vi "Main.vi"(11 "Module Admin":refnum<class "Delacor_lib_QMH_Module Admin.lvclass">) -> ()   [LabVIEW 2024, in "MoneyControl.lvlib"]
doc: "This template is based off of the Queued Message Handler design pattern and the Queued Message Handler project template that ships with LabVIEW.\n\nThe main difference is that the queue is private to this module and communication between modules is performed via Broadcast and Request events.\n\nRequest events are wrapped in public API methods and are handled in the Event Handling Loop (EHL) of this VI. Any module can register for Broadcast events sent by this module. The EHL generates messages based on user interface actions.\n\nThe Message Handling Loop (MHL) processes messages generated by the EHL, or by other messages. The messages are string values, so new messages can be added easily to the Message Cases case structure in the MHL. Each message cluster can also provide an optional value for Message Data, which is a variant that can be converted to whatever message-specific data is required.\n_____\nBased on DQMH Dev Tools: Project Template 7.1.0.1503."
uses:
  MoneyControl.lvlib
  <vilib>/Delacor/Delacor QMH/Libraries/Module Admin_class/Delacor_lib_QMH_Module Admin.lvclass
  Module Data--cluster.ctl
  <vilib>/Utility/miscctls.llb/LVFontTypeDef.ctl
  Stop Argument--cluster.ctl
  <vilib>/Delacor/Delacor QMH/Libraries/Message Queue_class/Delacor_lib_QMH_Message Queue.lvclass/Delacor_lib_QMH_Message Queue.ctl
  <vilib>/Delacor/Delacor QMH/Libraries/Module Admin_class/Delacor_lib_QMH_Module Admin.lvclass/Delacor_lib_QMH_Module Admin.ctl
  Draw FP in Subpanel Argument--cluster.ctl
  Remove From Subpanel Argument--cluster.ctl
  Incrementa Credito Argument--cluster.ctl
  Cancelar Argument--cluster.ctl
  <vilib>/Delacor/Delacor QMH/Libraries/Message Queue_class/Delacor_lib_QMH_Enqueue Message (Single).vi
  <vilib>/Delacor/Delacor QMH/Libraries/Module Admin_class/Delacor_lib_QMH_Get External Launch.vi
  <vilib>/Delacor/Delacor QMH/Libraries/Message Queue_class/Delacor_lib_QMH_Message Queue.lvclass
  <vilib>/PantherLAB/Message Module/Libraries/Message/PantherLAB_lib_Message.lvlib
panel:
  in  "Moneda 1":bool caption="1"
  in  "Moneda 5":bool caption="5"
  in  "Moneda 2":bool caption="2"
  out "error out":errorcluster
  out "Status":string
  in  "Moneda 10":bool caption="10"
  in  "Cancelar":bool
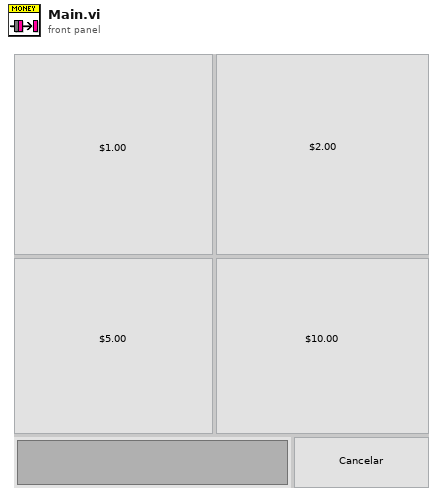
[diagram p1: front panel]
types:
  T1 = typedef "MoneyControl.lvlib/Request Events--cluster.ctl" = cluster{"Stop Module":refnum<user-event>, "Show Panel":refnum<user-event>, "Hide Panel":refnum<user-event>, "Get Module Execution Status":refnum<user-event>, "Show Diagram":refnum<user-event>, "Draw FP in Subpanel":refnum<user-event>, "Remove From Subpanel":refnum<user-event>, "Incrementa Credito":refnum<user-event>, "Cancelar":refnum<user-event>}
  T2 = typedef "PantherLAB_lib_Message.lvlib/Broadcast Events--cluster.ctl" = cluster{"Module Did Init":refnum<user-event>, "Status Updated":refnum<user-event>, "Error Reported":refnum<user-event>, "Module Did Stop":refnum<user-event>, "Update Module Execution Status":refnum<user-event>}
  T3 = typedef "MoneyControl.lvlib/Module Data--cluster.ctl" = cluster{"Status":string, "Sub Panel":refnum<vi>, "Credito":dbl}
  T4 = typedef "LVFontTypeDef.ctl" = cluster{"Font Name":string, "Size":u16, "Bold":bool, "Italic":bool, "Underline":bool, "Strikeout":bool, "Color":u32}
  T5 = enum32{"invalid lock state", "Not Locked", "Locked (No Password)", "Password-protected"}
  T6 = typedef "MoneyControl.lvlib/Stop Argument--cluster.ctl" = cluster{"Origin":string, "Exit via Stop Module Req?":bool, "Wait for Module to stop?":bool}
  T7 = typedef "MoneyControl.lvlib/Draw FP in Subpanel Argument--cluster.ctl" = cluster{"Sub Panel":refnum<vi>}
  T8 = typedef "MoneyControl.lvlib/Remove From Subpanel Argument--cluster.ctl" = cluster{"Boolean":bool}
  T9 = typedef "MoneyControl.lvlib/Incrementa Credito Argument--cluster.ctl" = cluster{"Credito":dbl}
  T10 = typedef "MoneyControl.lvlib/Cancelar Argument--cluster.ctl" = cluster{"Boolean":bool}
  T11 = enum32{"Invalid", "Standard", "Closed", "Hidden", "Minimized", "Maximized"}
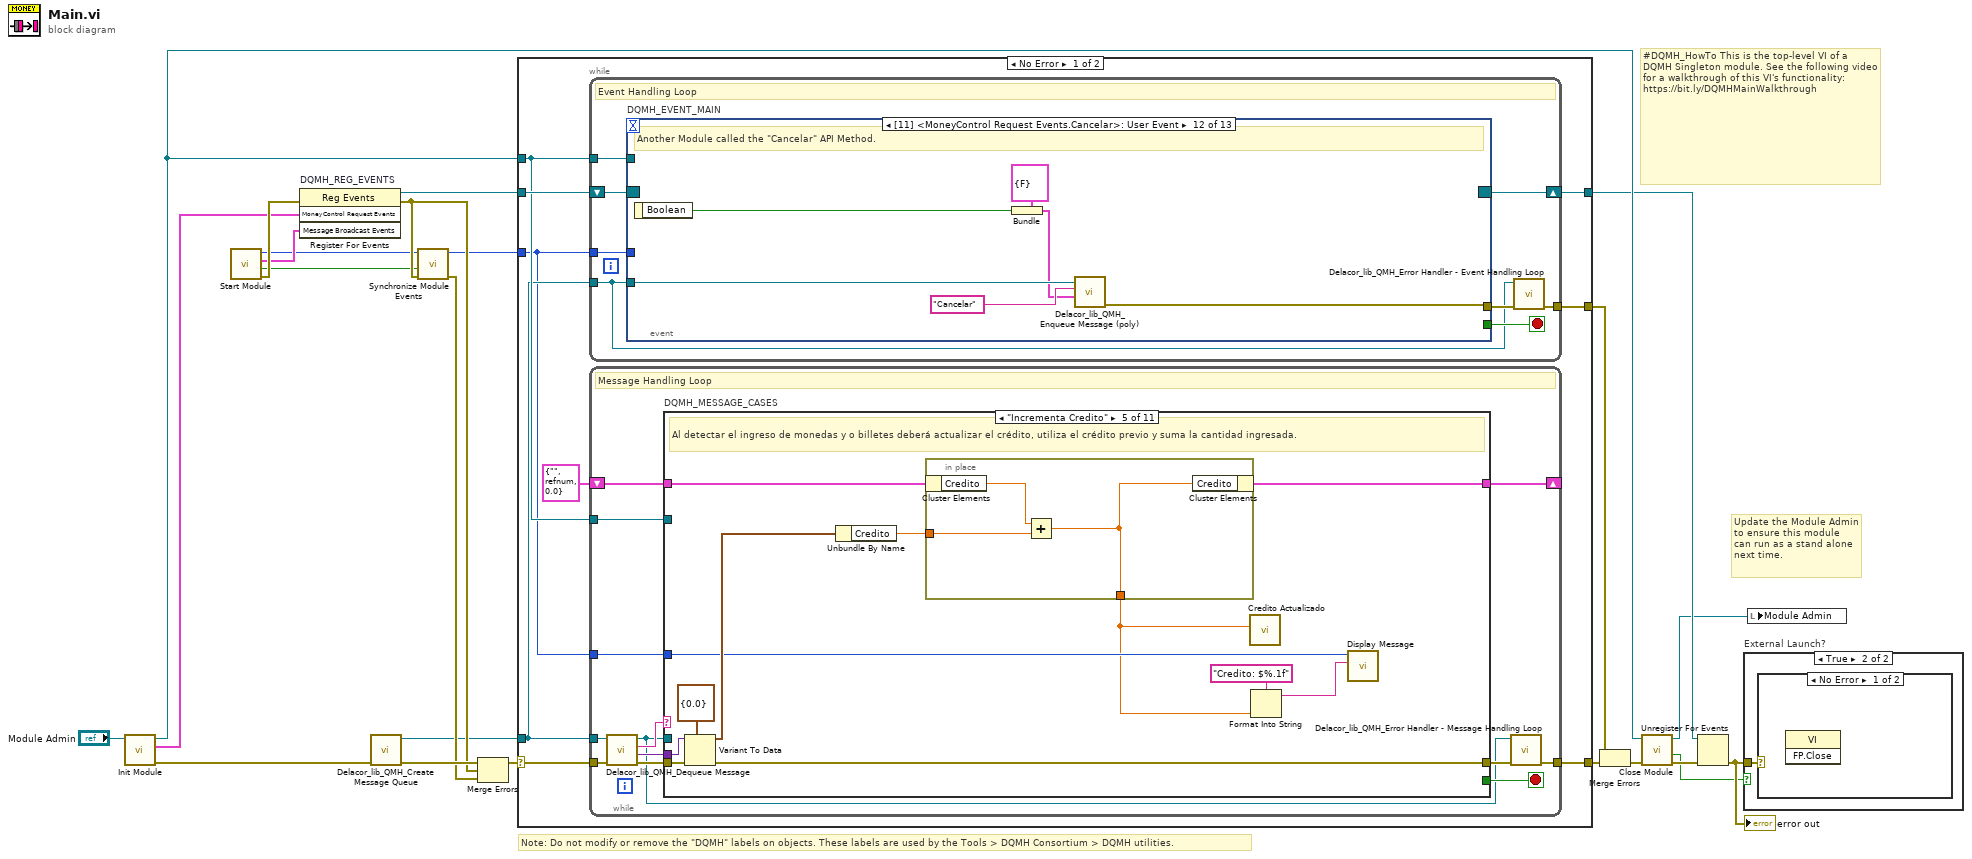
[diagram p0: block diagram]
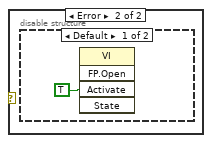
[diagram p3: hidden frame]
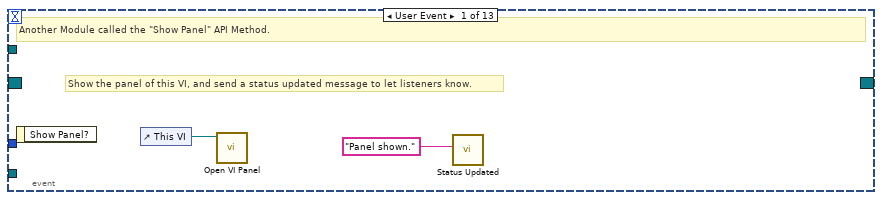
[diagram p5: hidden frame]
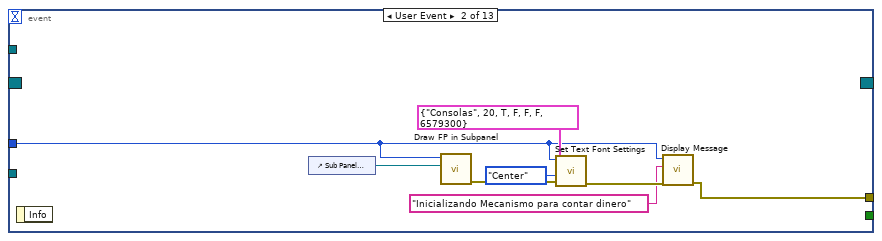
[diagram p6: hidden frame]
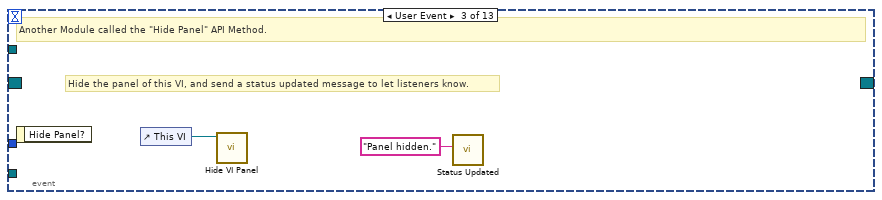
[diagram p7: hidden frame]
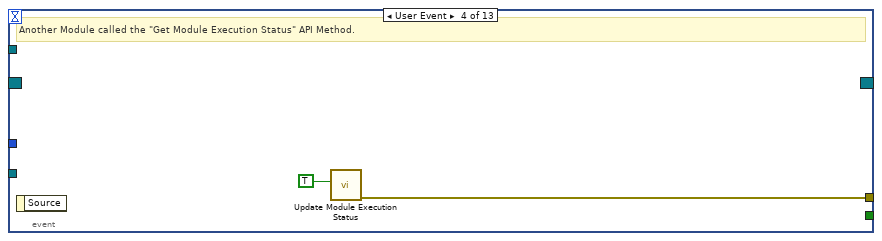
[diagram p8: hidden frame]
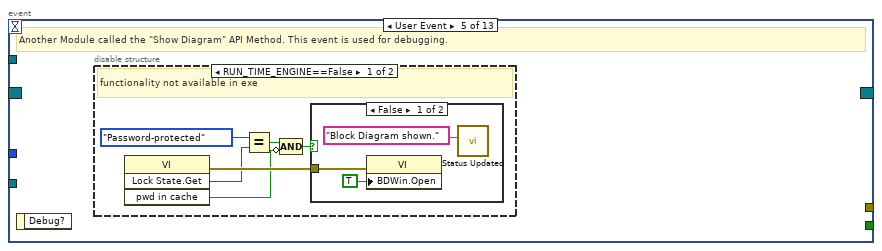
[diagram p9: hidden frame]
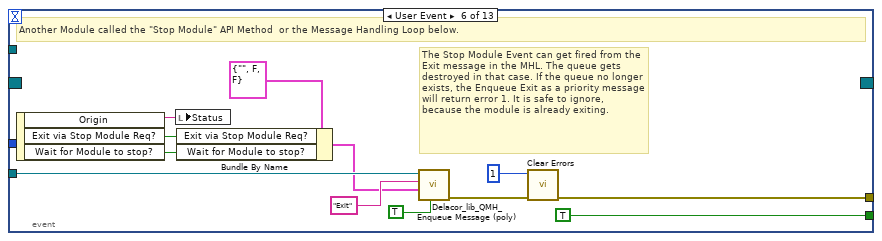
[diagram p12: hidden frame]
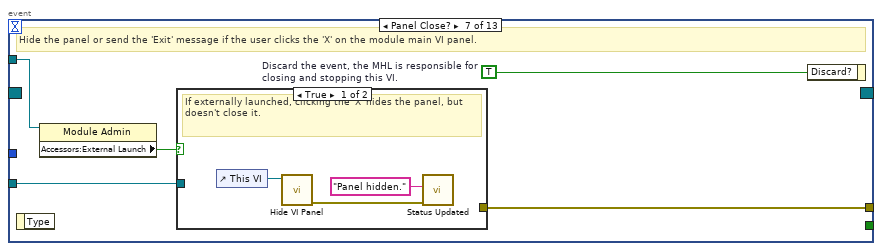
[diagram p13: hidden frame]
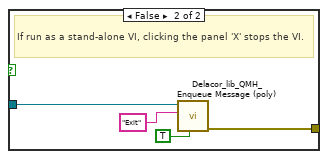
[diagram p14: hidden frame]
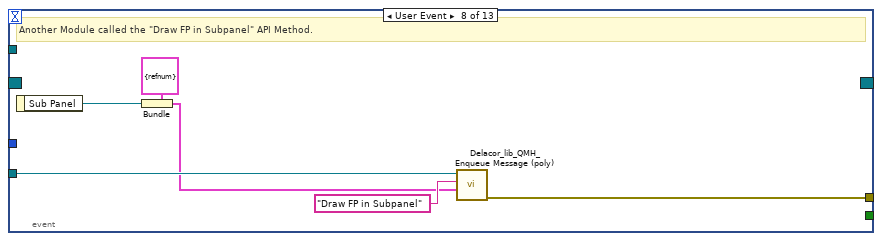
[diagram p15: hidden frame]
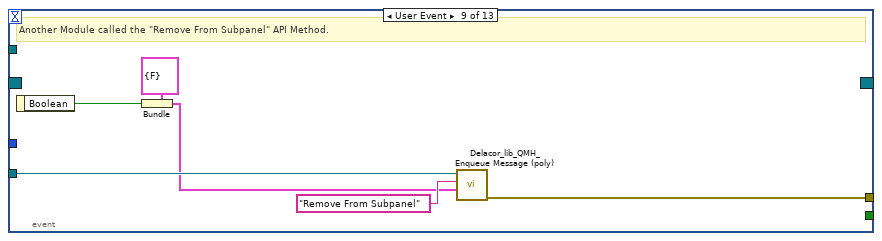
[diagram p16: hidden frame]
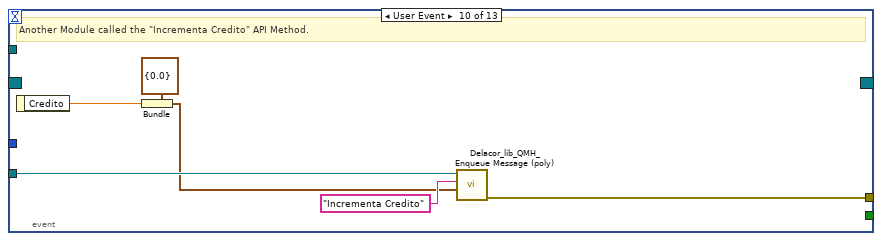
[diagram p17: hidden frame]
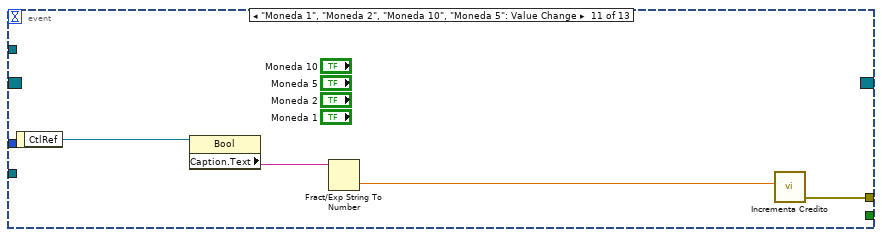
[diagram p18: hidden frame]
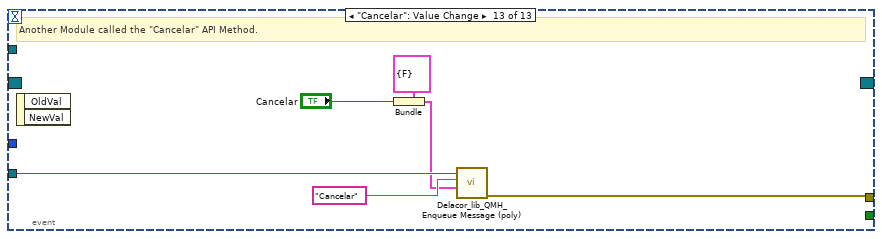
[diagram p19: hidden frame]
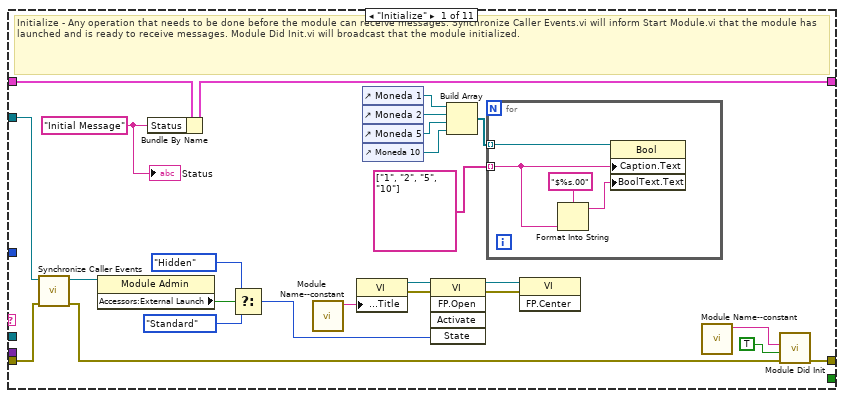
[diagram p20: hidden frame]
diagram:
  # "#DQMH_HowTo This is the top-level VI of a DQMH Singleton module. See the following video for a walkthrough of this VI's functionality: https://bit.ly/DQMHMainWalkthrough"
  # "Note: Do not modify or remove the \"DQMH\" labels on objects. These labels are used by the Tools > DQMH Consortium > DQMH utilities."
  # "Update the Module Admin to ensure this module can run as a stand alone next time."
  n1 = call "Init Module.vi"("Singleton Module Admin in"="Module Admin") -> ("error out"=w22:errorcluster, "MoneyControl Request Events"=w9:T1, "Singleton Module Admin out"=w12:refnum<class "Delacor_lib_QMH_Module Admin.lvclass">)  [unwired: 8 in]
  n2 = call <vilib>:"Start Module.vi"() -> ("error out"=w13:errorcluster, "Wait for Event Sync?"=w2:bool, "Message Broadcast Events"=w4:T2, "Module ID"=w3:i32)  [unwired: 7 in, 1 out]
  n3 = register-events "DQMH_REG_EVENTS"(error in=w13, w9, w4) -> (reference out=w10:refnum<event-registration>, error out=w15:errorcluster)  [unwired: 1 in]
  n4 = call <vilib>:"Delacor_lib_QMH_Create Message Queue.vi"("error in"=w22) -> ("error out"=w17:errorcluster, "Message Queue"=w8:refnum<class "Delacor_lib_QMH_Message Queue.lvclass">)  [unwired: 9 in]
  n5 = call <vilib>:"Synchronize Module Events.vi"("error in"=w15, "Wait for Event Sync?"=w2, "Module ID in"=w3) -> ("error out"=w14:errorcluster, "Module ID out"=w1:i32)  [unwired: 7 in]
  n6 = Merge Errors(w17, w15, w14) -> (w16:errorcluster)
  n7 = case shown="No Error" w16 {
    selector: w16 -> [w30 w292]
    tunnel: [w32 w291] -> w23
    tunnel: [w29 w290] -> w11
    tunnel: w10 -> [w27 w290]
    tunnel: w8 -> [w25 w286]
    tunnel: [w31 _] -> w20
    tunnel: w12 -> [w26 w287]
    tunnel: w1 -> [w24 w284]
    frame No Error {
      n8 = while {
        tunnel: w25 -> [w34]
        shift-right: [w37] -> w29
        shift-left: w27 -> [w38]
        tunnel: [w39] -> w31
        tunnel: w26 -> [w35]
        tunnel: w24 -> [w33]
        stop <- w36 stop-if-true
        # "Event Handling Loop"
        n9 = event "DQMH_EVENT_MAIN" shown="[11] <MoneyControl Request Events.Cancelar>: User Event" {
          selector: w38 -> [_ _ _ _ _ _ _ _ _ _ _ _ _]
          dyn-events: [_ _ _ _ _ _ _ _ _ _ _ _ _] -> w37
          timeout: _ -> [_ _ _ _ _ _ _ _ _ _ _ _ _]
          tunnel: [_ _ _ _ _ TRUE ("Discard?") _ _ _ _ _ _ _] -> w36
          tunnel: w34 -> [_ _ _ _ _ w71 w78 w92 w98 w104 _ w115 w121]
          tunnel: [_ w48 _ w54 _ w74 w80 w93 w99 w105 w109 w110 w117] -> w40
          tunnel: w35 -> [_ _ _ _ _ _ w77 _ _ _ _ _ _]
          tunnel: w33 -> [_ w44 _ _ _ _ _ _ _ _ _ _ _]
          event User Event {
            # "Show the panel of this VI, and send a status updated message to let listeners know."
            # "Another Module called the \"Show Panel\" API Method."
            n10 = event-data() -> ()  [unwired: 1 in, 1 out]
            n11 = control-ref of="This VI"() -> (w42:refnum<vi>)
            n12 = call "Open VI Panel.vi"("VI"=w42) -> ()  [unwired: 10 in, 1 out]
            n13 = call "Status Updated.vi"("Status"="Panel shown." ("format string")) -> ()  [unwired: 10 in, 1 out]
          }
          event User Event {
            n14 = event-data() -> ()  [unwired: 1 in, 1 out]
            n15 = control-ref of="Sub Panel Mensajes"() -> (w47:refnum<vi>)
            n16 = call <vilib>:"Draw FP in Subpanel.vi"("Sub Panel"=w47, "Module ID"=w44) -> ("error out"=w50:errorcluster)  [unwired: 9 in]
            n17 = call <vilib>:"Set Text Font Settings.vi"("error in"=w50, "Text.Justification"=enum16{"Left", "Center", "Right"}."Center", "Font"=T4 {"Font Name"="Consolas", "Size"=20, "Bold"=TRUE, "Italic"=FALSE, "Underline"=FALSE, "Strikeout"=FALSE, "Color"=6579300}, "Module ID"=w44) -> ("error out"=w49:errorcluster)  [unwired: 7 in]
            n18 = call <vilib>:"Display Message.vi"("error in"=w49, "Message"="Inicializando Mecanismo para contar dinero", "Module ID"=w44) -> ("error out"=w48:errorcluster)  [unwired: 8 in]
          }
          event User Event {
            # "Hide the panel of this VI, and send a status updated message to let listeners know."
            # "Another Module called the \"Hide Panel\" API Method."
            n19 = event-data() -> ()  [unwired: 1 in, 1 out]
            n20 = control-ref of="This VI"() -> (w52:refnum<vi>)
            n21 = call "Hide VI Panel.vi"("VI"=w52) -> ()  [unwired: 10 in, 1 out]
            n22 = call "Status Updated.vi"("Status"="Panel hidden." ("format string")) -> ()  [unwired: 10 in, 1 out]
          }
          event User Event {
            # "Another Module called the \"Get Module Execution Status\" API Method."
            n23 = event-data() -> ()  [unwired: 1 in, 1 out]
            n24 = call "Update Module Execution Status.vi"("Running?"=TRUE) -> ("error out"=w54:errorcluster)  [unwired: 10 in]
          }
          event User Event {
            # "Another Module called the \"Show Diagram\" API Method. This event is used for debugging."
            n25 = event-data() -> ()  [unwired: 1 in, 1 out]
            n26 = disable-structure shown="RUN_TIME_ENGINE==False" {
              frame condition #0 (active) {
                # "functionality not available in exe"
                n27 = invoke on="Invoke Node" class="VI" method="Lock State.Get"() -> (error out=w60:errorcluster, "Get Lock State"=w59:T5, "pwd in cache"=w56:bool)  [unwired: 4 in, 1 out]
                n28 = Equal?(x=T5."Password-protected", y=w59) -> (x = y?=w57:bool)
                n29 = Compound Arithmetic op=AND(w57, invert w56) -> (w55:bool)
                n30 = case shown="False" w55 {
                  tunnel: w60 -> [w63 _]
                  frame False {
                    n31 = property on="Property Node" class="VI"(error in=w63, "BDWin.Open"=TRUE ("Block Diagram Window:Open")) -> ()  [unwired: 1 in, 2 out]
                    n32 = call "Status Updated.vi"("Status"="Block Diagram shown." ("format string")) -> ()  [unwired: 10 in, 1 out]
                  }
                  frame True {
                    # "Password-protected VI, and the password is not in the cache. Do not show the diagram."
                  }
                }
              }
              frame condition #1 {
              }
            }
          }
          event User Event {
            # "The Stop Module Event can get fired from the Exit message in the MHL. The queue gets destroyed in that case. If the queue no longer exists, the Enqueue Exit as a priority message will return error 1. It is safe to ignore, because the module is already exiting."
            # "Another Module called the \"Stop Module\" API Method  or the Message Handling Loop below."
            n33 = event-data() -> ("Origin"=w70:string, "Exit via Stop Module Req?"=w66:bool, "Wait for Module to stop?"=w65:bool)  [unwired: 1 in]
            n34 = local write "Status"(w70) -> ()
            n35 = Bundle By Name(cluster=T6 {"Origin"="", "Exit via Stop Module Req?"=FALSE, "Wait for Module to stop?"=FALSE} ("Stop Argument"), "Exit via Stop Module Req?"=w66, "Wait for Module to stop?"=w65) -> (w64:T6)
            n36 = call-poly <vilib>:"Delacor_lib_QMH_Enqueue Message (poly).vi"("Priority Message? (F)"=TRUE, "Message Data"=w64, "Message"="Exit", "Message Queue in"=w71) -> ("error out"=w75:errorcluster)  [unwired: 6 in, 1 out]
            n37 = call <vilib>:"Clear Errors.vi"("error in (no error)"=w75, "specific error code to clear (0: all)"=1) -> ("error out"=w74:errorcluster)  [unwired: 4 in, 1 out]
          }
          event Panel Close? {
            w79 = TRUE  # Discard the event, the MHL is responsible for closing and stopping this VI.
            # "Hide the panel or send the 'Exit' message if the user clicks the 'X' on the module main VI panel."
            n38 = event-data() -> ()  [unwired: 1 in, 1 out]
            n39 = property on="Property Node" class="Module Admin"(reference=w77) -> ("Accessors:External Launch"=w76:bool)  [unwired: 1 in, 2 out]
            n40 = case shown="True" w76 {
              tunnel: w78 -> [_ w86]
              tunnel: [_ w87] -> w80
              frame True {
                # "If externally launched, clicking the 'X' hides the panel, but doesn't close it."
                n41 = control-ref of="This VI"() -> (w82:refnum<vi>)
                n42 = call "Hide VI Panel.vi"("VI"=w82) -> ("error out"=w83:errorcluster)  [unwired: 10 in]
                n43 = call "Status Updated.vi"("error in"=w83, "Status"="Panel hidden." ("format string")) -> ()  [unwired: 9 in, 1 out]
              }
              frame False {
                # "If run as a stand-alone VI, clicking the panel 'X' stops the VI."
                n44 = call-poly <vilib>:"Delacor_lib_QMH_Enqueue Message (poly).vi"("Priority Message? (F)"=TRUE, "Message"="Exit", "Message Queue in"=w86) -> ("error out"=w87:errorcluster)  [unwired: 7 in, 1 out]
              }
            }
            n45 = event-data ("Event Filter Node")("Discard?"=w79) -> ()  [unwired: 1 in, 1 out]
          }
          event User Event {
            # "Another Module called the \"Draw FP in Subpanel\" API Method."
            n46 = event-data() -> ("Sub Panel"=w88:refnum<vi>)  [unwired: 1 in]
            n47 = Bundle(cluster=T7 {"Sub Panel"=refnum} ("Draw FP in Subpanel Argument"), "Sub Panel"=w88) -> (w89:T7)
            n48 = call-poly <vilib>:"Delacor_lib_QMH_Enqueue Message (poly).vi"("Message Data"=w89, "Message"="Draw FP in Subpanel", "Message Queue in"=w92) -> ("error out"=w93:errorcluster)  [unwired: 7 in, 1 out]
          }
          event User Event {
            # "Another Module called the \"Remove From Subpanel\" API Method."
            n49 = event-data() -> ("Boolean"=w94:bool)  [unwired: 1 in]
            n50 = Bundle(cluster=T8 {"Boolean"=FALSE} ("Remove From Subpanel Argument"), "Boolean"=w94) -> (w95:T8)
            n51 = call-poly <vilib>:"Delacor_lib_QMH_Enqueue Message (poly).vi"("Message Data"=w95, "Message"="Remove From Subpanel", "Message Queue in"=w98) -> ("error out"=w99:errorcluster)  [unwired: 7 in, 1 out]
          }
          event User Event {
            # "Another Module called the \"Incrementa Credito\" API Method."
            n52 = event-data() -> ("Credito"=w100:dbl)  [unwired: 1 in]
            n53 = Bundle(cluster=T9 {"Credito"=0.0} ("Incrementa Credito Argument"), "Credito"=w100) -> (w101:T9)
            n54 = call-poly <vilib>:"Delacor_lib_QMH_Enqueue Message (poly).vi"("Message Data"=w101, "Message"="Incrementa Credito", "Message Queue in"=w104) -> ("error out"=w105:errorcluster)  [unwired: 7 in, 1 out]
          }
          event "Moneda 1", "Moneda 2", "Moneda 10", "Moneda 5": Value Change {
            n55 = event-data() -> ("CtlRef"=w108:refnum<vi>)  [unwired: 1 in]
            n56 = property class="Bool"(reference=w108) -> ("Caption.Text"=w107:string)  [unwired: 1 in, 2 out]
            n57 = Fract/Exp String To Number(string=w107) -> (number=w106:dbl)  [unwired: 3 in, 1 out]
            n58 = call "Incrementa Credito.vi"("Credito"=w106) -> ("error out"=w109:errorcluster)  [unwired: 10 in]
          }
          event User Event {
            # "Another Module called the \"Cancelar\" API Method."
            n59 = event-data() -> ("Boolean"=w111:bool)  [unwired: 1 in]
            n60 = Bundle(cluster=T10 {"Boolean"=FALSE} ("Cancelar Argument"), "Boolean"=w111) -> (w112:T10)
            n61 = call-poly <vilib>:"Delacor_lib_QMH_Enqueue Message (poly).vi"("Message Data"=w112, "Message"="Cancelar", "Message Queue in"=w115) -> ("error out"=w110:errorcluster)  [unwired: 7 in, 1 out]
          }
          event "Cancelar": Value Change {
            # "Another Module called the \"Cancelar\" API Method."
            n62 = event-data() -> ()  [unwired: 1 in, 2 out]
            n63 = Bundle(cluster=T10 {"Boolean"=FALSE} ("Cancelar Argument"), "Boolean"="Cancelar") -> (w118:T10)
            n64 = call-poly <vilib>:"Delacor_lib_QMH_Enqueue Message (poly).vi"("Message Data"=w118, "Message"="Cancelar", "Message Queue in"=w121) -> ("error out"=w117:errorcluster)  [unwired: 7 in, 1 out]
          }
        }
        n65 = call-dynamic "Delacor_lib_QMH_Error Handler - Event Handling Loop.vi"("error in"=w40, "Message Queue in"=w34) -> ("dup error in"=w39:errorcluster)  [unwired: 8 in, 1 out]
      }
      n66 = while {
        tunnel: w25 -> [w123]
        shift-right: [w129] -> _
        shift-left: T3 {"Status"="", "Sub Panel"=refnum, "Credito"=0.0} ("Data Cluster") -> [w130]
        tunnel: w30 -> [w134]
        tunnel: [w132] -> w32
        tunnel: w26 -> [w125]
        tunnel: w24 -> [w122]
        stop <- w128 stop-if-true
        # "Message Handling Loop"
        n67 = call-dynamic "Delacor_lib_QMH_Dequeue Message.vi"("error in"=w134, "Message Queue in"=w123) -> ("error out"=w133:errorcluster, "Message Data"=w126:variant, "Message"=w127:string, "Message Queue out"=w124:refnum<class "Delacor_lib_QMH_Message Queue.lvclass">)  [unwired: 6 in]
        n68 = case "DQMH_MESSAGE_CASES" shown="\"Incrementa Credito\"" w127 {
          selector: w127 -> [_ _ _ _ _ _ _ _ _ _ w279]
          tunnel: w124 -> [_ _ _ _ _ _ _ _ w242 w267 _]
          tunnel: w133 -> [w157 w165 w181 w199 w217 w232 w237 w239 w250 w273 w282]
          tunnel: [w155 w165 w180 w197 w216 w231 w236 w239 w246 w268 w283] -> w131
          tunnel: w130 -> [w146 w164 w176 w193 w212 w227 w235 w238 w244 w259 w280]
          tunnel: [w145 w164 w172 w190 w211 w226 w235 w238 w244 w259 w280] -> w129
          tunnel: [_ _ _ _ _ _ _ _ _ w266 _] -> w128
          tunnel: w126 -> [_ _ w175 w196 w215 w230 _ _ w243 w265 _]
          tunnel: w125 -> [w147 _ _ _ _ _ _ _ w241 w260 _]
          tunnel: w122 -> [_ _ _ _ w209 w224 _ _ _ w257 _]
          frame "Initialize" {
            w141 = "Initial Message" ("Initial Message")
            # "Initialize - Any operation that needs to be done before the module can receive messages. Synchronize Caller Events.vi will inform Start Module.vi that the module has launched and is ready to receive messages. Module Did Init.vi will broadcast that the module initialized."
            n69 = call "Synchronize Caller Events.vi"("error in"=w157, "Singleton Module Admin in"=w147) -> ("error out"=w156:errorcluster, "Singleton Module Admin out"=w142:refnum<class "Delacor_lib_QMH_Module Admin.lvclass">)  [unwired: 8 in]
            n70 = property on="Property Node" class="Module Admin"(reference=w142) -> ("Accessors:External Launch"=w151:bool)  [unwired: 1 in, 2 out]
            n71 = Bundle By Name(cluster=w146, "Status"=w141) -> (w145:T3)
            n72 = Select(t=T11."Hidden" ("State"), s=w151, f=T11."Standard" ("State")) -> (s? t:f=w148:T11)
            n73 = call "Module Name--constant.vi"() -> ("Module Name"=w154:string)  [unwired: 11 in]
            n74 = property on="Property Node" class="VI"("Front Panel.Title"=w154) -> (reference out=w153:refnum<vi>, error out=w159:errorcluster)  [unwired: 2 in]
            n75 = control-ref of="Moneda 1"() -> (w140:refnum<vi>)
            n76 = control-ref of="Moneda 2"() -> (w139:refnum<vi>)
            n77 = control-ref of="Moneda 5"() -> (w138:refnum<vi>)
            n78 = control-ref of="Moneda 10"() -> (w137:refnum<vi>)
            n79 = invoke on="Invoke Node" class="VI" method="FP.Open"(reference=w153, error in=w159, "State"=w148) -> (reference out=w152:refnum<vi>, error out=w158:errorcluster)  [unwired: 2 in, 3 out]
            n80 = Build Array(w140, w139, w138, w137) -> (w136:refnum<vi>[])
            n81 = for {
              tunnel: w136 -> [w163] mode=indexing
              tunnel: string[] ["1", "2", "5", "10"] -> [w162] mode=indexing
              n82 = Format Into String(format string="$%s.00", w162) -> (resulting string=w161:string)  [unwired: 2 in, 1 out]
              n83 = property class="Bool"(reference=w163, "Caption.Text"=w162, "BoolText.Text"=w161) -> ()  [unwired: 1 in, 2 out]
            }
            n84 = invoke on="Invoke Node" class="VI" method="FP.Center"(reference=w152, error in=w158) -> ()  [unwired: 1 in, 3 out]
            n85 = call "Module Name--constant.vi"() -> ("Module Name"=w143:string)  [unwired: 11 in]
            n86 = call "Module Did Init.vi"("error in"=w156, "Initialized?"=TRUE, "Origin"=w143) -> ("error out"=w155:errorcluster)  [unwired: 8 in]
            "Status" <- w141
          }
          frame "---Module Specific---" {
            # "Separator -- The following cases handle messages specific to this Module."
          }
          frame "Draw FP in Subpanel" {
            # "Draw FP in Subpanel"
            n87 = Variant To Data(error in=w181, type=T7 {"Sub Panel"=refnum} ("Draw FP in Subpanel Argument"), Variant=w175) -> (data=w173:T7, error out=w179:errorcluster)
            n88 = Unbundle By Name(w173) -> ("Sub Panel"=w171:refnum<vi>)
            n89 = control-ref of="This VI"() -> (w168:refnum<vi>)
            n90 = property class="VI"(reference=w168, error in=w179) -> (reference out=w167:refnum<vi>, error out=w177:errorcluster, "FP.State"=w166:T11)
            n91 = case shown="\"Closed\"" w166 {
              tunnel: [w182 w185] -> w169
              tunnel: [w183 w187] -> w178
              tunnel: w177 -> [w183 w186]
              tunnel: w167 -> [w182 w184]
              frame "Closed" {
              }
              frame "Standard", Default {
                n92 = invoke class="VI" method="FP.Close"(reference=w184, error in=w186) -> (reference out=w185:refnum<vi>, error out=w187:errorcluster)  [unwired: 1 in, 1 out]
              }
            }
            n93 = invoke class="SubPnl" method="Insert VI"(reference=w171, error in=w178, "VI Ref"=w169) -> (reference out=w170:refnum<vi>, error out=w180:errorcluster)  [unwired: 1 in, 2 out]
            n94 = Bundle By Name(cluster=w176, "Sub Panel"=w170) -> (w172:T3)
          }
          frame "Remove From Subpanel" {
            # "Remove From Subpanel"
            n95 = Variant To Data(error in=w199, type=T8 {"Boolean"=FALSE} ("Remove From Subpanel Argument"), Variant=w196) -> (data=w194:T8, error out=w198:errorcluster)
            n96 = Unbundle By Name(w194) -> ()  [unwired: 1 out]
            n97 = Unbundle By Name(w193) -> ("Sub Panel"=w192:refnum<vi>)
            n98 = Not A Number/Path/Refnum?(number/path/refnum=w192) -> (NaN/Path/Refnum?=w191:bool)
            n99 = case shown="True" w191 {
              tunnel: w198 -> [w203 w205]
              tunnel: [w202 w205] -> w197
              tunnel: w192 -> [w201 _]
              tunnel: ["Module Removed from Subpanel" "This module has not been inserted into the subpanel"] -> w188
              frame False {
                n100 = invoke class="SubPnl" method="Remove VI"(reference=w201, error in=w203) -> (error out=w202:errorcluster)  [unwired: 1 in, 2 out]
              }
              frame True {
              }
            }
            n101 = Bundle By Name(cluster=w193, "Sub Panel"=refnum<vi> refnum) -> (w190:T3)
            n102 = call "Status Updated.vi"("Status"=w188) -> ()  [unwired: 10 in, 1 out]
          }
          frame "Incrementa Credito" {
            # "Al detectar el ingreso de monedas y o billetes deberá actualizar el crédito, utiliza el crédito previo y suma la cantidad ingresada."
            n103 = Variant To Data(error in=w217, type=T9 {"Credito"=0.0} ("Incrementa Credito Argument"), Variant=w215) -> (data=w213:T9, error out=w216:errorcluster)
            n104 = Unbundle By Name(w213) -> ("Credito"=w210:dbl)
            n105 = in-place {
              in-place-border: w210 -> [w219]
              in-place-border: [w218] -> w206
              n106 = in-place-cluster #1(w212) -> ("Credito"=w220:dbl)
              n107 = Add(x=w220, y=w219) -> (x+y=w218:dbl)
              n108 = in-place-cluster #1("Credito"=w218) -> (w211:T3)
            }
            n109 = call "Credito Actualizado.vi"("Credito"=w206) -> ()  [unwired: 10 in, 1 out]
            n110 = Format Into String(format string="Credito: $%.1f", w206) -> (resulting string=w208:string)  [unwired: 2 in, 1 out]
            n111 = call <vilib>:"Display Message.vi"("Message"=w208, "Module ID"=w209) -> ()  [unwired: 9 in, 1 out]
          }
          frame "Cancelar" {
            # "Regresa la totalidad del crédito actual"
            n112 = Variant To Data(error in=w232, type=T10 {"Boolean"=FALSE} ("Cancelar Argument"), Variant=w230) -> (data=w228:T10, error out=w231:errorcluster)
            n113 = Unbundle By Name(w228) -> ()  [unwired: 1 out]
            n114 = in-place {
              in-place-border: [w234] -> w225
              in-place-border: [w233] -> w222
              w234 = 0.0 ("Credito")
              n115 = in-place-cluster #2(w227) -> ("Credito"=w233:dbl)
              n116 = in-place-cluster #2("Credito"=w234) -> (w226:T3)
            }
            n117 = Format Into String(format string="Credito Regresado $%.1f, Vuelve Pronto", w222) -> (resulting string=w223:string)  [unwired: 2 in, 1 out]
            n118 = call <vilib>:"Display Message.vi"("Message"=w223, "Module ID"=w224) -> ()  [unwired: 9 in, 1 out]
            n119 = call "Credito Actualizado.vi"("Credito"=w225) -> ()  [unwired: 10 in, 1 out]
          }
          frame "---Copy This Frame---" {
            # "Duplicate this frame when creating new messages.  Change this comment in the duplicated frame to describe this message."
            n120 = Merge Errors(w237) -> (w236:errorcluster)
          }
          frame "---Exit and Error Handling---" {
            # "Separator - The following cases handle errors and exit messages."
          }
          frame "Error" {
            # "#DQMH_CodeRecommended - If the module is running in standalone mode (External Launch = FALSE), this code will pop up an error dialog and call the 'Exit' message if an error occurs. Add more fine-grained error management here."
            # "Error - Check the error message data and respond accordingly. This message is sent by the \"Error Handler\" VIs at the end of each loop in this application."
            n121 = property on="Property Node" class="Module Admin"(reference=w241) -> ("Accessors:External Launch"=w240:bool)  [unwired: 1 in, 2 out]
            n122 = Variant To Data(error in=w250, type=errorcluster {"status"=FALSE, "code"=0, "source"=""} ("error constant"), Variant=w243) -> (data=w245:errorcluster, error out=w248:errorcluster)
            n123 = local write "error out"(w245) -> ()
            n124 = call "Error Reported.vi"("Error"=w245) -> ()  [unwired: 10 in, 1 out]
            n125 = case shown="False" w240 {
              tunnel: [w255 _] -> w247
              tunnel: w242 -> [w253 _]
              tunnel: w245 -> [w254 _]
              frame False {
                n126 = disable-structure shown="Default" {
                  disable-tunnel: w254 -> [w256 _]
                  frame condition #0 (active) {
                    # "If the module is running standalone, then pop up an error dialog and call the \"Exit\" message."
                    n127 = call <vilib>:"Simple Error Handler.vi"("error in (no error)"=w256) -> ()  [unwired: 4 in, 5 out]
                  }
                  frame condition #1 {
                    # "To prevent the Simple Error Handler VI from being loaded (e.g. when deploying to a Real-Time target), add the Conditional Disable Symbol \"DQMH_Disable_SEH\" to your project and set it to TRUE."
                  }
                }
                n128 = call-poly <vilib>:"Delacor_lib_QMH_Enqueue Message (poly).vi"("Priority Message? (F)"=TRUE, "Message"="Exit", "Message Queue in"=w253) -> ("error out"=w255:errorcluster)  [unwired: 7 in, 1 out]
              }
              frame True {
                # "If the module was launched externally, calling the Error Reported broadcast VI is the only action performed by the \"Error\" message. The module's caller can then process the error appropriately."
              }
            }
            n129 = Merge Errors(w248, w247) -> (w246:errorcluster)
          }
          frame "Exit" {
            w264 = 91  # 91: not all Exit messages will have an argument
            w266 = TRUE  # Stop the VI
            # "Release the message queue reference"
            # "#DQMH_CodeNeeded - Add any required cleanup code here."
            # "Exit - Exit the application."
            n130 = Variant To Data(error in=w273, type=T6 {"Origin"="", "Exit via Stop Module Req?"=FALSE, "Wait for Module to stop?"=FALSE} ("Stop Argument"), Variant=w265) -> (data=w262:T6, error out=w270:errorcluster)
            n131 = call <vilib>:"Clear Errors.vi"("error in (no error)"=w270, "specific error code to clear (0: all)"=w264) -> ("error out"=w272:errorcluster)  [unwired: 4 in, 1 out]
            n132 = control-ref of="This VI"() -> (w261:refnum<vi>)
            n133 = call-dynamic "Delacor_lib_QMH_Release Message Queue.vi"("error in"=w272, "Message Queue"=w267) -> ("error out"=w271:errorcluster)  [unwired: 9 in]
            n134 = call "Handle Exit.vi"("Stop Argument"=w262, "Admin in"=w260, "VI reference"=w261) -> ("error out"=w269:errorcluster)  [unwired: 7 in, 1 out]
            n135 = Merge Errors(w271, w269) -> (w268:errorcluster)
            n136 = Unbundle By Name(w259) -> ("Sub Panel"=w258:refnum<vi>)
            n137 = call "Error Reported.vi"("Error"=w268) -> ()  [unwired: 10 in, 1 out]
            n138 = invoke class="SubPnl" method="Remove VI"(reference=w258) -> ()  [unwired: 2 in, 3 out]
            n139 = call <vilib>:"Stop Module.vi"("Module ID"=w257) -> ()  [unwired: 10 in, 1 out]
          }
          frame Default {
            # "'Default' case only runs if there is a message that isn't defined in any of the other cases.  Output a programming error."
            n140 = call "Module Name--constant.vi"() -> ("Module Name"=w278:string)  [unwired: 11 in]
            n141 = Format Into String(format string="The invalid message string \"%s\" was received in the Message Handling Loop for module \"%s\".", w279, w278) -> (resulting string=w274:string)  [unwired: 2 in, 1 out]
            n142 = call <vilib>:"Error Cluster From Error Code.vi"("show call chain? (False)"=TRUE, "error message (\"\")"=w274, "error code (0)"=1) -> ("error out"=w281:errorcluster)  [unwired: 6 in]
            n143 = Merge Errors(w282, w281) -> (w283:errorcluster)
          }
        }
        n144 = call-dynamic "Delacor_lib_QMH_Error Handler - Message Handling Loop.vi"("error in"=w131, "Message Queue in"=w124) -> ("dup error in"=w132:errorcluster)  [unwired: 8 in, 1 out]
      }
    }
    frame Error {
      # "Synchronize Caller Events.vi will inform Start Module.vi that the module has launched and will let the code calling Start Module.vi register for broadcasts and would permit the caller receive the broadcast that an error occurred at launch time."
      n145 = call-dynamic "Delacor_lib_QMH_Release Message Queue.vi"("error in"=w292, "Message Queue"=w286) -> ("error out"=w291:errorcluster)  [unwired: 9 in]
      n146 = call "Synchronize Caller Events.vi"("Singleton Module Admin in"=w287) -> ("error out"=w293:errorcluster)  [unwired: 9 in, 1 out]
      n147 = call "Module Name--constant.vi"() -> ("Module Name"=w289:string)  [unwired: 11 in]
      n148 = Format Into String(format string="An error occurred during initialization. %s is no longer running.", w289) -> (resulting string=w285:string)  [unwired: 2 in, 1 out]
      n149 = Merge Errors(w291, w293) -> (w294:errorcluster)
      n150 = call "Error Reported.vi"("Additional Information"=w285, "Error"=w294) -> ()  [unwired: 9 in, 1 out]
      n151 = call <vilib>:"Stop Module.vi"("Origin"=w285, "Module ID"=w284) -> ()  [unwired: 9 in, 1 out]
    }
  }
  n152 = Merge Errors(w20, w23) -> (w19:errorcluster)
  n153 = call "Close Module.vi"("error in"=w19, "Module Admin in"=w12) -> ("error out"=w21:errorcluster, "External Launch"=w5:bool, "Module Admin out"=w6:refnum<class "Delacor_lib_QMH_Module Admin.lvclass">)  [unwired: 7 in]
  n154 = Unregister For Events(event registration refnum=w11, error in=w21) -> (error out=w18:errorcluster)
  "error out" <- w18
  n155 = case "External Launch?" shown="True" w5 {
    tunnel: w18 -> [_ w295]
    frame False {
    }
    frame True {
      n156 = case shown="No Error" w295 {
        frame No Error {
          n157 = invoke on="Invoke Node" class="VI" method="FP.Close"() -> ()  [unwired: 3 in, 3 out]
        }
        frame Error {
          n158 = disable-structure shown="Default" {
            frame condition #0 (active) {
              n159 = invoke class="VI" method="FP.Open"("Activate"=TRUE ("Activate?")) -> ()  [unwired: 4 in, 5 out]
            }
            frame condition #1 {
              # "Don't show panel on error if running inside a built EXE."
            }
          }
        }
      }
    }
  }
  n160 = local write "Module Admin"(w6) -> ()
